vi "Read Name.vi"(8 "Error In":errorcluster, 11 "Tag In":refnum<class "Tag.lvclass">) -> (0 "Error Out":errorcluster, 2 "Name":string, 3 "Tag Out":refnum<class "Tag.lvclass">)   [LabVIEW 2017, in "Mustache.lvlib" / "Tokens.lvlib" / "Tag.lvclass"]
uses:
  Tag.lvclass
  Tag.lvclass/Tag.ctl
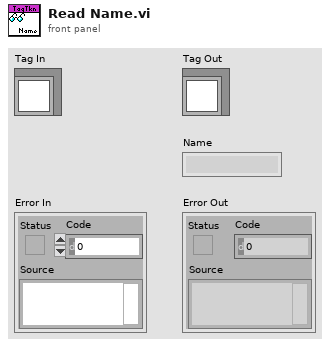
[diagram p1: front panel]
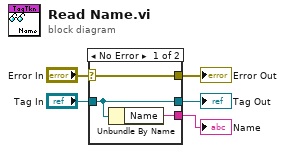
[diagram p0: block diagram]
diagram:
  n1 = case shown="No Error" "Error In" {
    selector: "Error In" -> [w8 w9]
    tunnel: [w8 w9] -> w4
    tunnel: [w7 w10] -> w2
    tunnel: "Tag In" -> [w7 w10]
    tunnel: [w6 _] -> w1
    frame No Error {
      n2 = Unbundle By Name(w7) -> ("Name"=w6:string)
    }
    frame Error {
    }
  }
  "Error Out" <- w4
  "Tag Out" <- w2
  "Name" <- w1
